vi "TestController.vi"() -> ()   [LabVIEW 2009]
panel:
  in  "STOP":bool
  in  "PROCESS":string
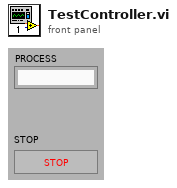
[diagram p1: front panel]
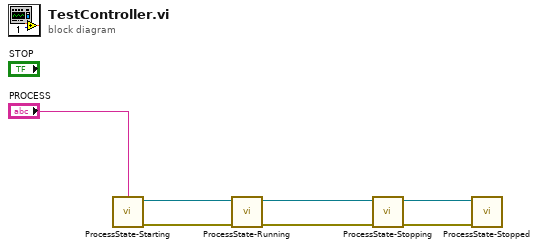
[diagram p0: block diagram]
diagram:
  n1 = call "ProcessState-Starting.vi"("PROCESS"="PROCESS") -> ("ProcessStateNotifier"=w3:refnum<notifier>, "error in (no error)"=w6:errorcluster)  [unwired: 1 in, 6 out]
  n2 = call "ProcessState-Running.vi"("ProcessStateNotifier in"=w3, "error in (no error)"=w6) -> ("ProcessStateNotifier out"=w2:refnum<notifier>, "error out"=w5:errorcluster)  [unwired: 6 out]
  n3 = call "ProcessState-Stopping.vi"("ProcessStateNotifier in"=w2, "error in (no error)"=w5) -> ("ProcessStateNotifier out"=w1:refnum<notifier>, "error out"=w4:errorcluster)  [unwired: 6 out]
  n4 = call "ProcessState-Stopped.vi"("ProcessStateNotifier in"=w1, "error in (no error)"=w4) -> ()  [unwired: 8 out]
